vi "Parse Param and ConPane Info.vi"(9 "VI ConPane":T3={"pattern"=4815, "terminals"=[]}, 10 "Method Params":T5[](array[typedef])) -> (1 "VI Input Builders":T1[](array[typedef]), 2 "CLFN Param Info":T2[](array[typedef]))   [LabVIEW 2014]
doc: "Copyright (c) 2016 Sze Howe Koh\n\nThis Source Code Form is subject to the terms of the Mozilla Public License, v. 2.0. If a copy of the MPL was not distributed with this file, You can obtain one at http://mozilla.org/MPL/2.0/."
uses:
  Data Structures/JSON/Param.ctl
  Data Structures/JSON/Connector Pane.ctl
  Data Structures/JSON/Connector Pane Terminal.ctl
  Data Structures/DLL Parameter Info.ctl
  Data Structures/VI Input Builder.ctl
  Param Writers/Abstract Param Writer/Abstract Param Writer.lvclass
  Param Writers/TypeConv/Action.ctl
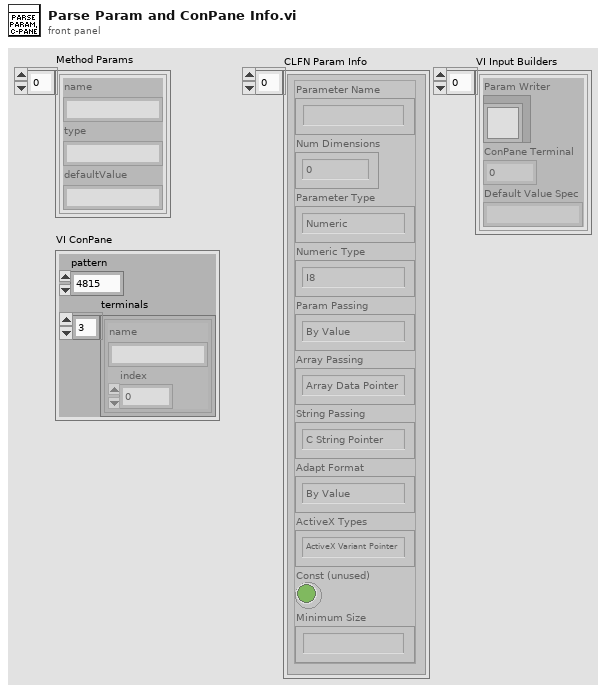
[diagram p1: front panel]
types:
  T1 = typedef "VI Input Builder.ctl" = cluster{"Param Writer":refnum<class "Abstract Param Writer.lvclass">, "ConPane Terminal":u32, "Default Value Spec":string}
  T2 = typedef "DLL Parameter Info.ctl" = cluster{"Parameter Name":string, "Num Dimensions":i32, "Parameter Type":enum16{"Numeric", "Array", "String", "Waveform", "Digital Waveform", "Digital Table", "ActiveX", "Any", "Instance Data Pointer", "Void"}, "Numeric Type":enum16{"I8", "I16", "I32", "I64", "U8", "U16", "U32", "U64", "SGL", "DBL", "PTR INT", "PTR UINT"}, "Param Passing":enum16{"By Value", "Pointer To Value"}, "Array Passing":enum16{"Array Data Pointer", "Array Handle", "Array Handle Pointer"}, "String Passing":enum16{"C String Pointer", "Pascal String Pointer", "String Handle", "String Handle Pointer"}, "Adapt Format":enum16{"By Value", "Pointer To Value"}, "ActiveX Types":enum16{"ActiveX Variant Pointer", "IDispatch* Pointer", "IUnknown* Pointer"}, "Const (unused)":bool, "Minimum Size":string}
  T3 = typedef "Connector Pane.ctl" = cluster{"pattern":u32, "terminals":T4[]}
  T4 = typedef "Connector Pane Terminal.ctl" = cluster{"name":string, "index":u32}
  T5 = typedef "Param.ctl" = cluster{"name":string, "type":string, "defaultValue":string}
  T6 = typedef "Action.ctl" = enum16{"Register Type", "Register Projection", "Obtain Writer", "Get Projection", "Get Type Path", "Get Type Category"}
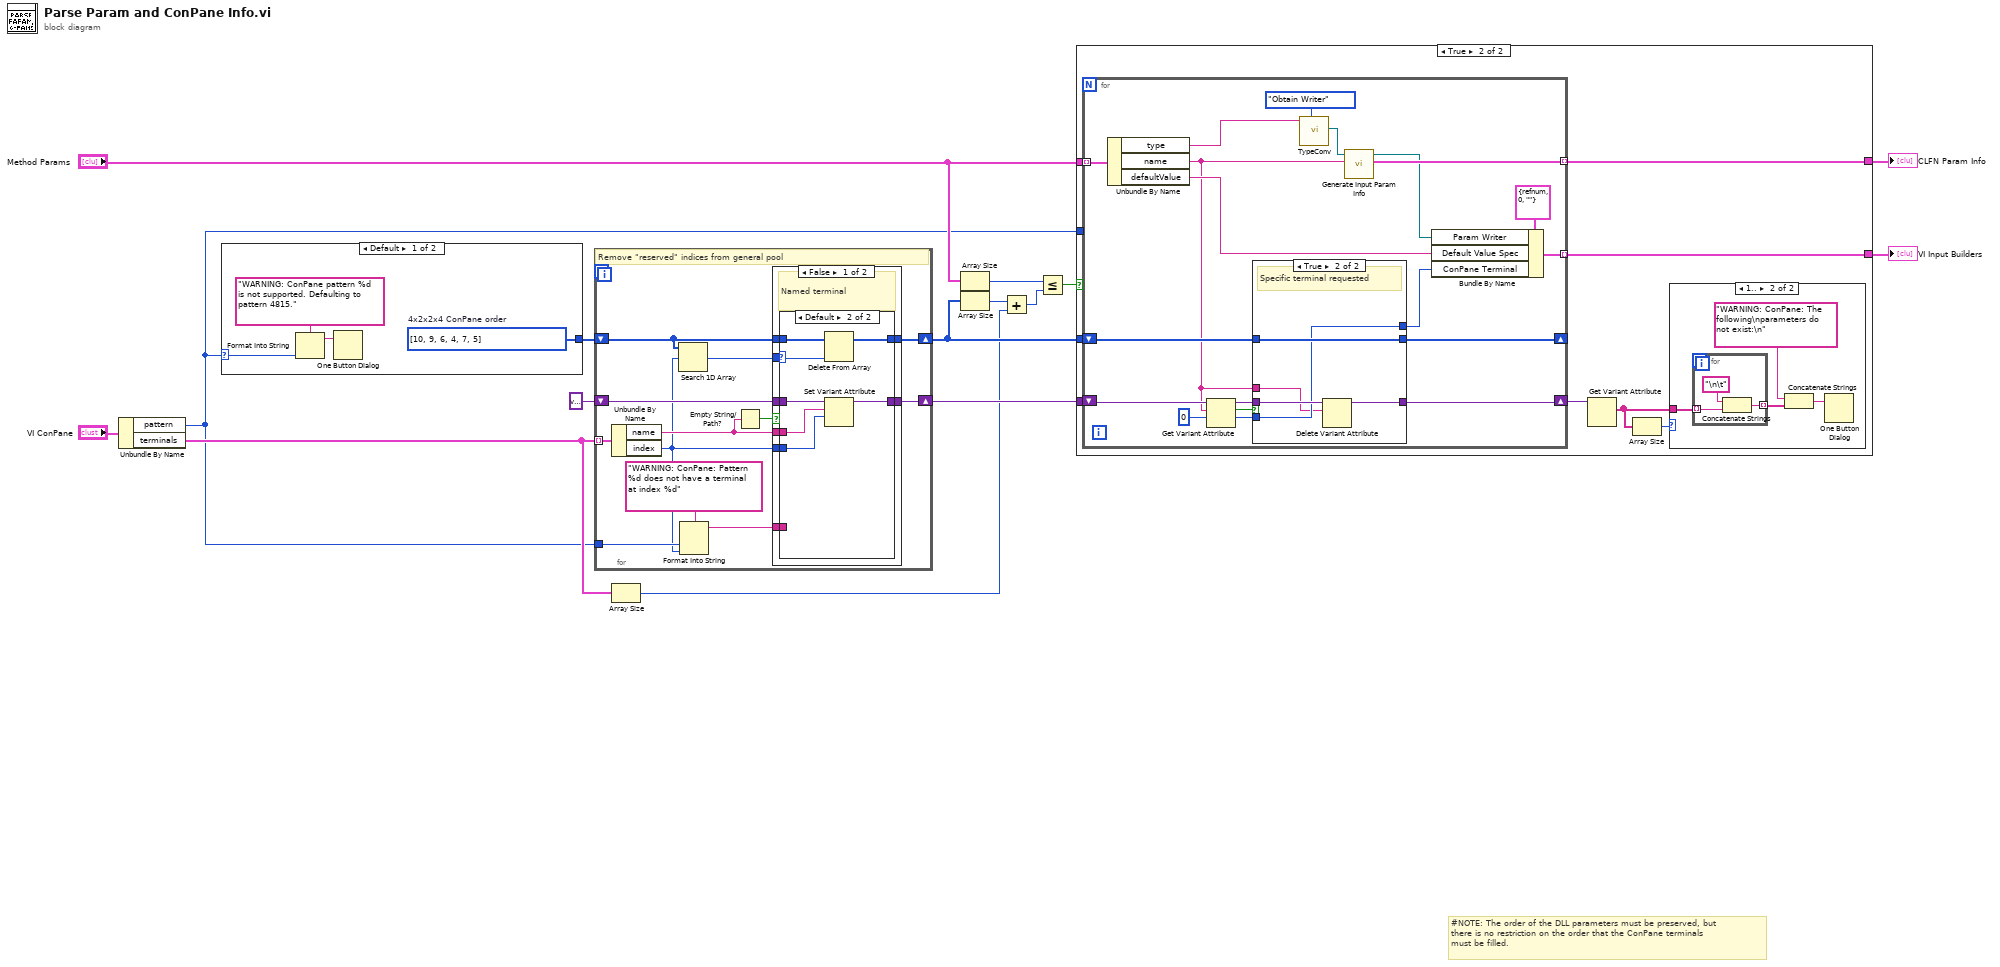
[diagram p0: block diagram]
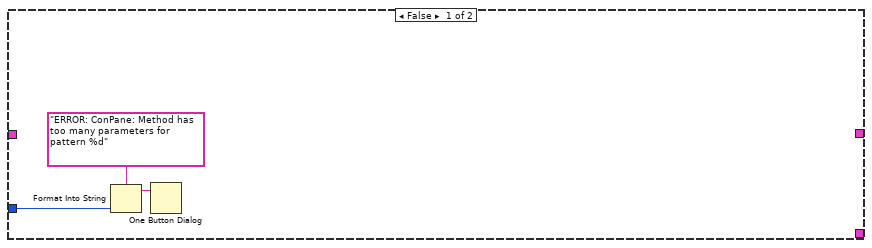
[diagram p2: hidden frame]
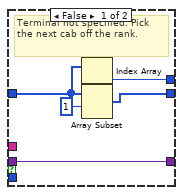
[diagram p4: hidden frame]
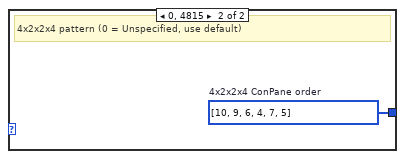
[diagram p5: hidden frame]
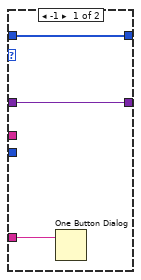
[diagram p6: hidden frame]
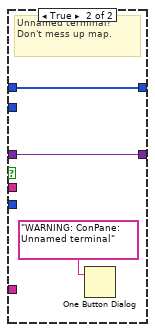
[diagram p7: hidden frame]
diagram:
  # "#NOTE: The order of the DLL parameters must be preserved, but\nthere is no restriction on the order that the ConPane terminals \nmust be filled."
  n1 = Unbundle By Name("VI ConPane") -> ("pattern"=w1:u32, "terminals"=w5:T4[])
  n2 = case shown="Default" w1 {
    selector: w1 -> [w18 _]
    tunnel: [w16 w20] -> w8
    frame Default {
      w16 = u32[] [10, 9, 6, 4, 7, 5]  # 4x2x2x4 ConPane order
      n3 = Format Into String(format string="WARNING: ConPane pattern %d is not supported. Defaulting to pattern 4815." ("message"), w18) -> (resulting string=w17:string)  [unwired: 2 in, 1 out]
      n4 = One Button Dialog(message=w17) -> ()  [unwired: 1 in, 1 out]
    }
    frame 0, 4815 {
      w20 = u32[] [10, 9, 6, 4, 7, 5]  # 4x2x2x4 ConPane order
      # "4x2x2x4 pattern (0 = Unspecified, use default)"
    }
  }
  n5 = for {
    tunnel: w5 -> [w32] mode=indexing
    shift-right: [w28] -> w6
    shift-left: variant ("Variant") -> [w29]
    shift-right: [w27] -> w7
    shift-left: w8 -> [w26]
    tunnel: w1 -> [w23]
    # "Remove \"reserved\" indices from general pool"
    n6 = Unbundle By Name(w32) -> ("name"=w30:string, "index"=w22:u32)
    n7 = Search 1D Array(1D array=w26, element=w22) -> (index of element=w25:i32)  [unwired: 1 in]
    n8 = Format Into String(format string="WARNING: ConPane: Pattern %d does not have a terminal at index %d", w23, w22) -> (resulting string=w21:string)  [unwired: 2 in, 1 out]
    n9 = Empty String/Path?(string/path=w30) -> (empty?=w31:bool)
    n10 = case shown="False" w31 {
      tunnel: w30 -> [w34 _]
      tunnel: w29 -> [w33 w52]
      tunnel: w22 -> [w35 _]
      tunnel: [w36 w52] -> w28
      tunnel: [w39 w51] -> w27
      tunnel: w26 -> [w40 w51]
      tunnel: w25 -> [w38 _]
      tunnel: w21 -> [w37 _]
      frame False {
        # "Named terminal"
        n11 = case shown="Default" w38 {
          selector: w38 -> [_ w48]
          tunnel: w40 -> [w42 w50]
          tunnel: [w42 w49] -> w39
          tunnel: w37 -> [w43 _]
          tunnel: [w41 w46] -> w36
          tunnel: w33 -> [w41 w47]
          tunnel: w35 -> [_ w45]
          tunnel: w34 -> [_ w44]
          frame -1 {
            n12 = One Button Dialog(message=w43) -> ()  [unwired: 1 in, 1 out]
          }
          frame Default {
            n13 = Delete From Array(array=w50, index=w48) -> (array with subset deleted=w49:u32[])  [unwired: 1 in, 1 out]
            n14 = Set Variant Attribute(Variant=w47, name=w44, value=w45) -> (Variant out=w46:variant)  [unwired: 1 in, 2 out]
          }
        }
      }
      frame True {
        # "Unnamed terminal!\nDon't mess up map."
        n15 = One Button Dialog(message="WARNING: ConPane: Unnamed terminal") -> ()  [unwired: 1 in, 1 out]
      }
    }
  }
  n16 = Array Size(array=w5) -> (size(s)=w4:i32)
  n17 = Array Size(array="Method Params") -> (size(s)=w13:i32)
  n18 = Array Size(array=w7) -> (size(s)=w3:i32)
  n19 = Add(x=w3, y=w4) -> (x+y=w2:i32)
  n20 = Less Or Equal?(x=w13, y=w2) -> (x <= y?=w9:bool)
  n21 = case shown="True" w9 {
    tunnel: w6 -> [_ w64]
    tunnel: w7 -> [_ w63]
    tunnel: "Method Params" -> [_ w62]
    tunnel: [_ w61] -> w11
    tunnel: [_ w60] -> w10
    tunnel: w1 -> [w54 _]
    frame False {
      n22 = Format Into String(format string="ERROR: ConPane: Method has too many parameters for pattern %d", w54) -> (resulting string=w56:string)  [unwired: 2 in, 1 out]
      n23 = One Button Dialog(message=w56) -> ()  [unwired: 1 in, 1 out]
    }
    frame True {
      n24 = for {
        tunnel: w62 -> [w90] mode=indexing
        tunnel: [w84] -> w61 mode=indexing
        shift-right: [w83] -> _
        shift-left: w63 -> [w75]
        tunnel: [w79] -> w60 mode=indexing
        shift-right: [w77] -> w59
        shift-left: w64 -> [w89]
        n25 = Unbundle By Name(w90) -> ("type"=w85:string, "name"=w72:string, "defaultValue"=w80:string)
        n26 = Get Variant Attribute(Variant=w89, name=w72, default value (empty Variant)=u32 0 ("index")) -> (duplicate Variant=w78:variant, found=w73:bool, value=w74:u32)  [unwired: 1 in, 1 out]
        n27 = case shown="True" w73 {
          tunnel: w75 -> [w94 w100]
          tunnel: w74 -> [_ w97]
          tunnel: [w95 w97] -> w76
          tunnel: [w93 w100] -> w83
          tunnel: w78 -> [w91 w99]
          tunnel: [w91 w98] -> w77
          tunnel: w72 -> [_ w96]
          frame False {
            # "Terminal not specified. Pick\nthe next cab off the rank."
            n28 = Index Array(array=w94) -> (element=w95:u32)  [unwired: 1 in]
            n29 = Array Subset(array=w94, index=1) -> (w93:u32[])  [unwired: 1 in]
          }
          frame True {
            # "Specific terminal requested"
            n30 = Delete Variant Attribute(6:w96, 7:w99) -> (3:w98:variant)  [unwired: 1 in, 2 out]
          }
        }
        n31 = call "TypeConv.vi"("Action"=Action."Obtain Writer", "Type Name"=w85) -> ("Param Writer"=w87:refnum<class "Abstract Param Writer.lvclass">)  [unwired: 5 in, 4 out]
        n32 = call-dynamic "Generate Input Param Info.vi"("Param Name"=w72, "Abstract Param Writer in"=w87) -> ("Param Info"=w84:T2, "Abstract Param Writer out"=w81:refnum<class "Abstract Param Writer.lvclass">)  [unwired: 8 in]
        n33 = Bundle By Name(cluster=T1 {"Param Writer"=refnum, "ConPane Terminal"=0, "Default Value Spec"=""}, "Param Writer"=w81, "Default Value Spec"=w80, "ConPane Terminal"=w76) -> (w79:T1)
      }
      n34 = Get Variant Attribute(Variant=w59) -> (names=w58:string[])  [unwired: 3 in, 3 out]
      n35 = Array Size(array=w58) -> (size(s)=w57:i32)
      n36 = case shown="1.." w57 {
        tunnel: w58 -> [_ w68]
        frame ..0 {
        }
        frame 1.. {
          n37 = for {
            tunnel: w68 -> [w71] mode=indexing
            tunnel: [w69] -> w67 mode=indexing
            n38 = Concatenate Strings("\n\t" ("string"), w71) -> (w69:string)
          }
          n39 = Concatenate Strings("WARNING: ConPane: The following\nparameters do not exist:\n", w67) -> (w65:string)
          n40 = One Button Dialog(message=w65) -> ()  [unwired: 1 in, 1 out]
        }
      }
    }
  }
  "CLFN Param Info" <- w11
  "VI Input Builders" <- w10
